vi "Elapsed Time.vi"(8 "Error In":errorcluster, 11 "Timer Handle":T1) -> (0 "Error Out":errorcluster, 1 "Time Elapsed":bool, 2 "Elapsed Time":dbl, 3 "Timer Handle":T1)   [LabVIEW 2016, in "Timer Session.lvclass"]
doc: "Returns the time that has elapsed in the timer after the last reset/obtaining the timer.\n\nYou can specify the input as timer name or timer reference. Using reference executes faster."
uses:
  Timer Session.lvclass
  Typedefs/Session Handle.ctl
  Timer Session.lvclass/Timer Session.ctl
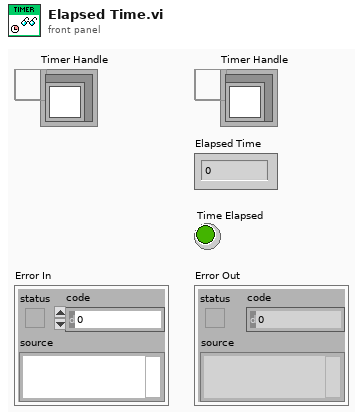
[diagram p1: front panel]
types:
  T1 = typedef "Timer Session.lvclass/Session Handle.ctl" = refnum<data-value>
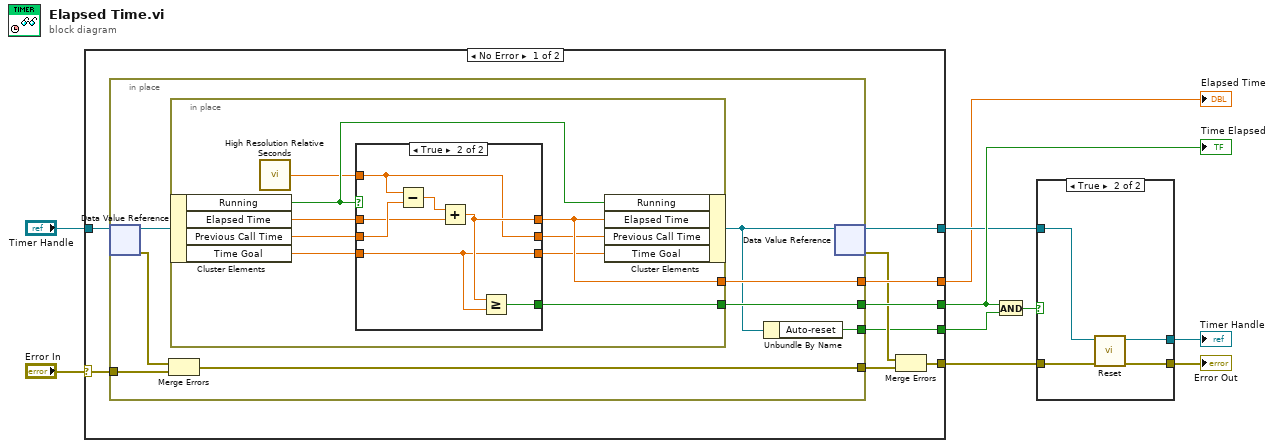
[diagram p0: block diagram]
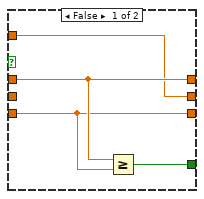
[diagram p2: hidden frame]
diagram:
  n1 = case shown="No Error" "Error In" {
    selector: "Error In" -> [w12 w49]
    tunnel: [w19 _] -> w7
    tunnel: [w18 _] -> w1
    tunnel: [w15 w49] -> w8
    tunnel: "Timer Handle" -> [w17 w48]
    tunnel: [w16 w48] -> w4
    tunnel: [w11 _] -> w6
    frame No Error {
      n2 = in-place {
        in-place-border: [w27] -> w19
        in-place-border: [w26] -> w18
        in-place-border: [w24] -> w13
        in-place-border: w12 -> [w22]
        in-place-border: [w20] -> w11
        n3 = in-place-dvr #1(w17) -> (w25:refnum<class "Timer Session.lvclass">, w23:errorcluster)
        n4 = Merge Errors(w23, w22) -> (w24:errorcluster)
        n5 = in-place {
          in-place-border: [w35] -> w27
          in-place-border: [w33] -> w26
          n6 = in-place-cluster #2(w25) -> ("Running"=w32:bool, "Elapsed Time"=w34:dbl, "Previous Call Time"=w31:dbl, "Time Goal"=w36:dbl)
          n7 = call <vilib>:"High Resolution Relative Seconds.vi"() -> ("relative seconds"=w28:dbl)
          n8 = case shown="True" w32 {
            tunnel: w31 -> [_ w47]
            tunnel: w36 -> [w39 w43]
            tunnel: [w38 w46] -> w35
            tunnel: w34 -> [w40 w45]
            tunnel: [w40 w44] -> w33
            tunnel: [w37 w41] -> w30
            tunnel: [w39 w43] -> w29
            tunnel: w28 -> [w37 w41]
            frame False {
              n9 = Greater Or Equal?(x=w40, y=w39) -> (x >= y?=w38:bool)
            }
            frame True {
              n10 = Subtract(x=w41, y=w47) -> (x-y=w42:dbl)
              n11 = Add(x=w42, y=w45) -> (x+y=w44:dbl)
              n12 = Greater Or Equal?(x=w44, y=w43) -> (x >= y?=w46:bool)
            }
          }
          n13 = in-place-cluster #2("Running"=w32, "Elapsed Time"=w33, "Previous Call Time"=w30, "Time Goal"=w29) -> (w21:refnum<class "Timer Session.lvclass">)
        }
        n14 = Unbundle By Name(w21) -> ("Auto-reset"=w20:bool)
        n15 = in-place-dvr #1(w21) -> (w16:T1, w14:errorcluster)
      }
      n16 = Merge Errors(w14, w13) -> (w15:errorcluster)
    }
    frame Error {
    }
  }
  "Time Elapsed" <- w7
  "Elapsed Time" <- w1
  n17 = And(x=w7, y=w6) -> (x .and. y?=w5:bool)
  n18 = case shown="True" w5 {
    tunnel: w8 -> [w50 w55]
    tunnel: w4 -> [w51 w54]
    tunnel: [w50 w53] -> w3
    tunnel: [w51 w52] -> w2
    frame False {
    }
    frame True {
      n19 = call "Reset.vi"("Error In"=w55, "Timer Handle"=w54) -> ("Error Out"=w53:errorcluster, "Timer Handle"=w52:T1)  [unwired: 8 in]
    }
  }
  "Timer Handle" <- w2
  "Error Out" <- w3
